vi "Update Outputs (Speed Controlled).vi"() -> ()   [LabVIEW 2012]
uses:
  Robot Global Data.vi
  <vilib>/addons/control/pid/NI_PID_pid.lvlib
  <vilib>/Rock Robotics/WPI/Solenoid/WPI_SolenoidSetEnum.vi
  <vilib>/Rock Robotics/WPI/Solenoid/WPI_SolenoidValue.ctl
  <vilib>/Rock Robotics/WPI/RobotDrive/WPI_RobotDriveArcadeDrive_Standard(NoSaturation).vi
  <vilib>/addons/control/pid/pid.llb/PID (DBL).vi
panel:
  out "Loop Time 2":u32(graph)
  out "Right Distance (ft)":dbl
  out "Left Distance (ft)":dbl
  out "Right Rate":dbl(graph)
  out "Left Rate":dbl(graph)
  in  "Shooter Speed (no encoder)":dbl(slide)=0.5 scale=0.0..1.0
  in  "Reset?":bool
  out "Shooter Output":dbl
  out "Loop Time":u32
  out "Rate":dbl
  out "Wheel Rate":dbl(graph)
  in  "Bang-Bang Output Range":T1={"Maximum"=1.0, "Minimum (Probably 0)"=0.0}
  in  "Bang-Bang Deadband Size":dbl=1.0
  in  "PID Output Range":cluster{"output high":dbl, "output low":dbl}={"output high"=1.0, "output low"=0.0} {"output low" format="%.2f"; "output high" format="%.2f"}
  in  "Shooter PID Gains":T2={"proportional gain (Kc)"=1.0, "integral time (Ti, min)"=0.01, "derivative time (Td, min)"=0.0} {"derivative time (Td, min)" format="%.3f"; "integral time (Ti, min)" format="%.3f"; "proportional gain (Kc)" format="%.3f"}
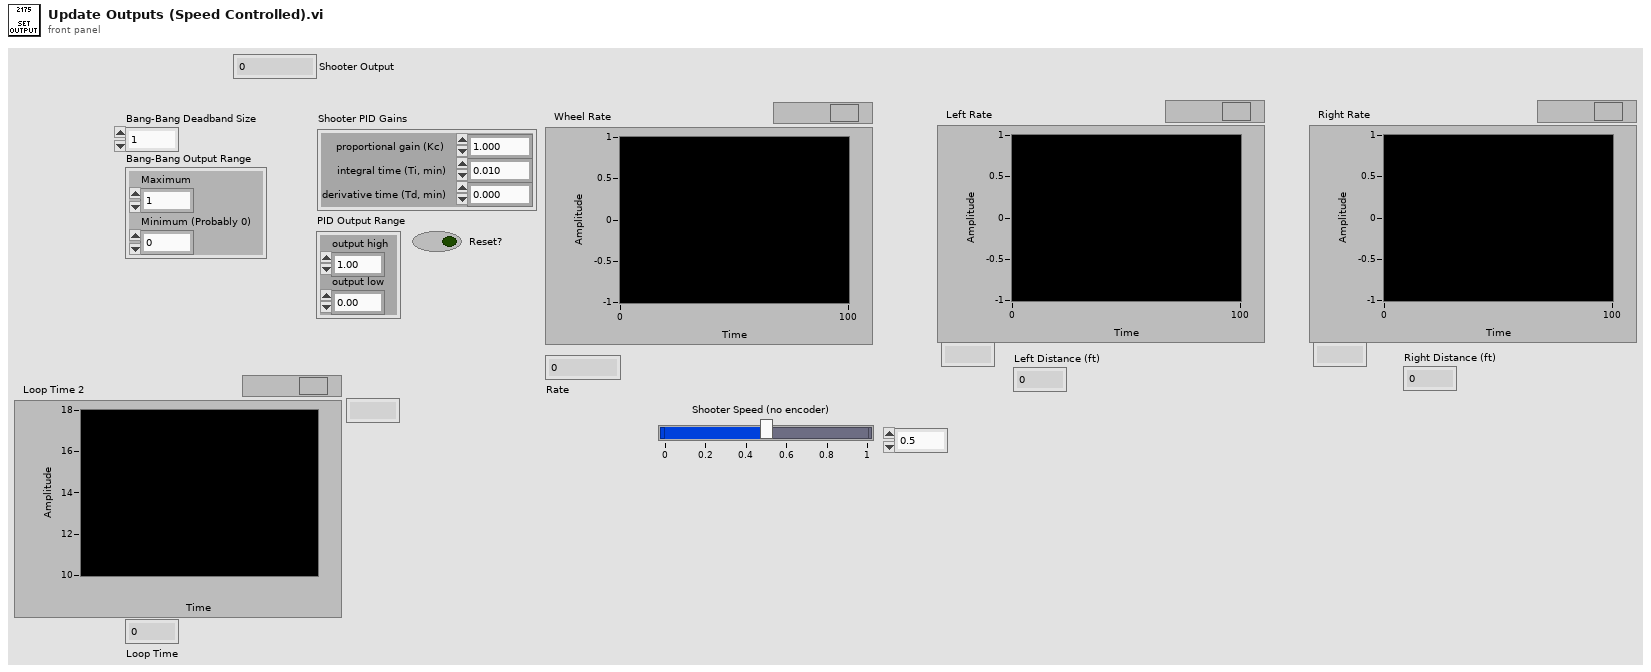
[diagram p1: front panel]
types:
  T1 = cluster{"Maximum":dbl, "Minimum (Probably 0)":dbl}
  T2 = cluster{"proportional gain (Kc)":dbl, "integral time (Ti, min)":dbl, "derivative time (Td, min)":dbl}
  T3 = typedef "WPI_SolenoidDevRef.ctl" = cluster{"DevStatus":errorcluster, "Solenoid Module":T4, "Forward Solenoid Channel":T5, "Reverse Solenoid Channel":T5}
  T4 = typedef "FPGA_TypedefSolenoidModule.ctl" = enum16{"Solenoid Module 1", "Solenoid Module 2"}
  T5 = typedef "WPI_SolenoidChannel.ctl" = enum8{"Solenoid 1", "Solenoid 2", "Solenoid 3", "Solenoid 4", "Solenoid 5", "Solenoid 6", "Solenoid 7", "Solenoid 8", "Invalid"}
  T6 = typedef "WPI_RobotDriveDevRef.ctl" = cluster{"DevStatus":errorcluster, "Motors[]":T7[], "Square Inputs":bool, "Max Output":dbl, "Isochronous":bool}
  T7 = typedef "WPI_MotorControlDeviceRef.ctl" = cluster{"DeviceStatus":errorcluster, "Type":enum16{"PWM", "CAN"}, "PWM":cluster{"Digital Module":T8, "PWM Channel":T9, "DeadBand":T10}, "CAN":cluster{"Device Number":u8, "Control Mode":T11, "Semaphore":T12, "Max Vout":dbl}, "Invert":bool, "TransformRef":T13, "InvTransformRef":T13}
  T8 = typedef "FPGA_TypedefDigitalModule.ctl" = enum16{"Digital Module 1", "Digital Module 2"}
  T9 = typedef "FPGA_DIOPWMChannel.ctl" = enum8{"PWM 1", "PWM 2", "PWM 3", "PWM 4", "PWM 5", "PWM 6", "PWM 7", "PWM 8", "PWM 9", "PWM 10", "Invalid"}
  T10 = typedef "WPI_PWMDeadband.ctl" = cluster{"Name":string, "maxPositivePwm":i32, "minPositivePwm":i32, "centerPwm":i32, "maxNegativePwm":i32, "minNegativePwm":i32, "angularRange":u16}
  T11 = typedef "WPI_CANJaguar_ControlMode.ctl" = enum8{"Percent VBus", "Current", "Speed", "Position", "Voltage"}
  T12 = typedef "Semaphore RefNum" = refnum<k1>
  T13 = typedef "WPI_PWMTransform_ConPane.ctl" = refnum<vi>
  T14 = typedef "WPI_DigitalInputDevRef.ctl" = cluster{"DevStatus":errorcluster, "DIO Channel":T15, "Digital Module":T8}
  T15 = typedef "FPGA_DIOChannel.ctl" = enum8{"DIO 1", "DIO 2", "DIO 3", "DIO 4", "DIO 5", "DIO 6", "DIO 7", "DIO 8", "DIO 9", "DIO 10", "DIO 11", "DIO 12", "DIO 13", "DIO 14", "Invalid"}
  T16 = typedef "WPI_EncoderDevRef.ctl" = cluster{"DevStatus":errorcluster, "EncoderIndex":T17, "CounterIndex":T18, "DistancePerCount":dbl, "Decoding Type":T19}
  T17 = typedef "FPGA_EncoderIdx.ctl" = enum8{"Enc 0", "Enc 1", "Enc 2", "Enc 3", "Invalid"}
  T18 = typedef "FPGA_CounterCtrSystemIndex.ctl" = enum8{"Ctr 0", "Ctr 1", "Ctr 2", "Ctr 3", "Ctr 4", "Ctr 5", "Ctr 6", "Ctr 7", "Invalid"}
  T19 = typedef "WPI_EncoderType.ctl" = enum16{"1x", "2x", "4x"}
  T20 = typedef "WPI_SolenoidValue.ctl" = enum16{"Off", "On", "Forward", "Reverse"}
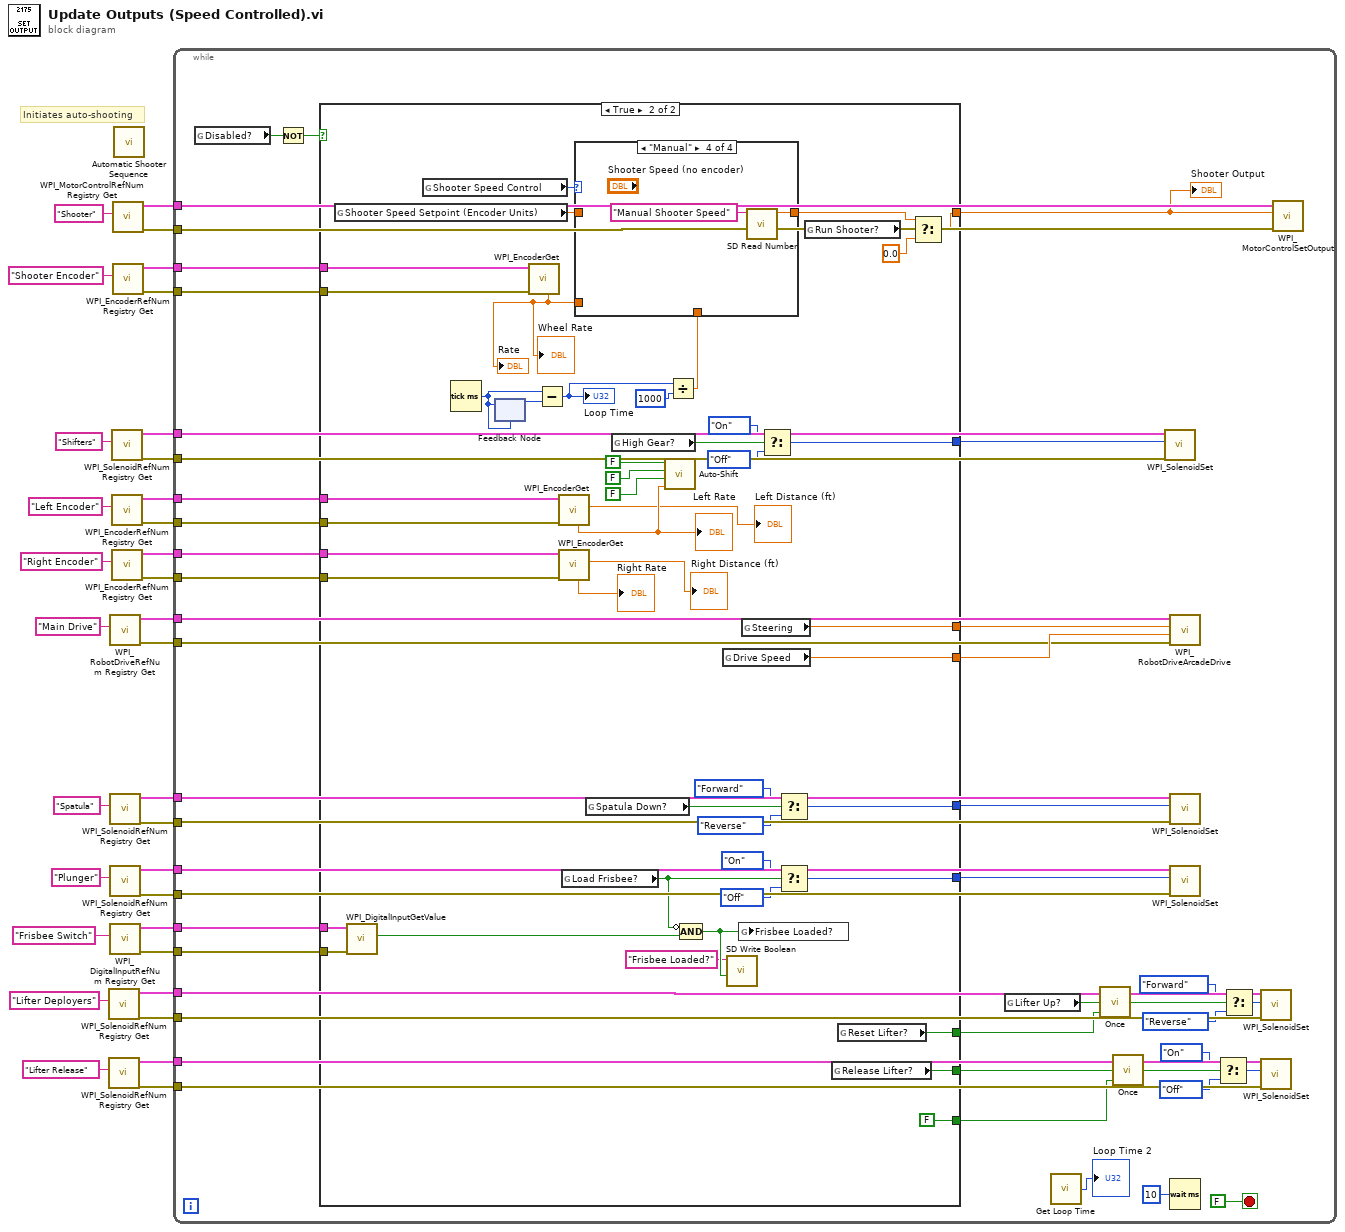
[diagram p0: block diagram]
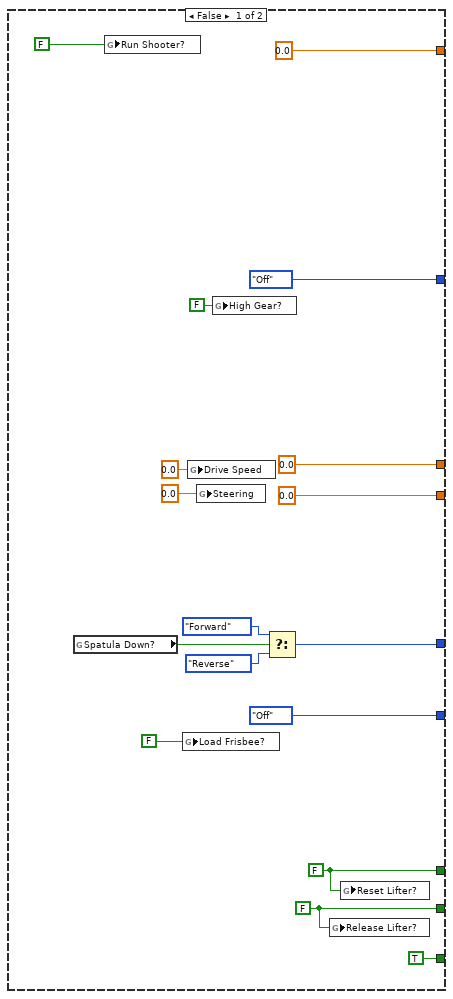
[diagram p2: hidden frame]
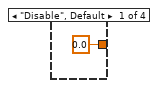
[diagram p3: hidden frame]
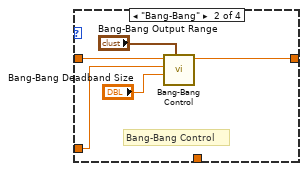
[diagram p4: hidden frame]
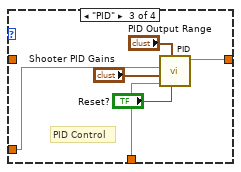
[diagram p5: hidden frame]
diagram:
  # "Initiates auto-shooting"
  n1 = call <vilib>:"WPI_SolenoidRefNum Registry Get.vi"("refnum name"="Lifter Deployers") -> ("error out"=w4:errorcluster, "SolenoidDevRef"=w5:T3)  [unwired: 9 in]
  n2 = call <vilib>:"WPI_SolenoidRefNum Registry Get.vi"("refnum name"="Lifter Release") -> ("error out"=w3:errorcluster, "SolenoidDevRef"=w2:T3)  [unwired: 9 in]
  n3 = call <vilib>:"WPI_RobotDriveRefNum Registry Get.vi"("refnum name"="Main Drive") -> ("error out"=w25:errorcluster, "RobotDriveDevRef"=w26:T6)  [unwired: 9 in]
  n4 = call <vilib>:"WPI_SolenoidRefNum Registry Get.vi"("refnum name"="Spatula") -> ("error out"=w19:errorcluster, "SolenoidDevRef"=w20:T3)  [unwired: 9 in]
  n5 = call <vilib>:"WPI_SolenoidRefNum Registry Get.vi"("refnum name"="Plunger") -> ("error out"=w18:errorcluster, "SolenoidDevRef"=w17:T3)  [unwired: 9 in]
  n6 = call <vilib>:"WPI_DigitalInputRefNum Registry Get.vi"("refnum name"="Frisbee Switch") -> ("error out"=w7:errorcluster, "DigitalInputDevRef"=w8:T14)  [unwired: 9 in]
  n7 = call <vilib>:"WPI_SolenoidRefNum Registry Get.vi"("refnum name"="Shifters") -> ("error out"=w22:errorcluster, "SolenoidDevRef"=w23:T3)  [unwired: 9 in]
  n8 = call <vilib>:"WPI_EncoderRefNum Registry Get.vi"("refnum name"="Left Encoder") -> ("error out"=w13:errorcluster, "EncoderDevRef"=w14:T16)  [unwired: 9 in]
  n9 = call <vilib>:"WPI_EncoderRefNum Registry Get.vi"("refnum name"="Right Encoder") -> ("error out"=w12:errorcluster, "EncoderDevRef"=w11:T16)  [unwired: 9 in]
  n10 = call <vilib>:"WPI_MotorControlRefNum Registry Get.vi"("refnum name"="Shooter") -> ("error out"=w28:errorcluster, "MotorControlDevRef"=w29:T7)  [unwired: 9 in]
  n11 = call <vilib>:"WPI_EncoderRefNum Registry Get.vi"("refnum name"="Shooter Encoder") -> ("error out"=w30:errorcluster, "EncoderDevRef"=w31:T16)  [unwired: 9 in]
  n12 = call "Automatic Shooter Sequence.vi"() -> ()  [unwired: 12 in]
  n13 = while {
    tunnel: w31 -> [w74]
    tunnel: w30 -> [w73]
    tunnel: w29 -> [w72]
    tunnel: w28 -> [w71]
    tunnel: w26 -> [w68]
    tunnel: w25 -> [w67]
    tunnel: w23 -> [w66]
    tunnel: w22 -> [w65]
    tunnel: w20 -> [w62]
    tunnel: w19 -> [w63]
    tunnel: w17 -> [w61]
    tunnel: w18 -> [w60]
    tunnel: w14 -> [w56]
    tunnel: w13 -> [w55]
    tunnel: w11 -> [w53]
    tunnel: w12 -> [w54]
    tunnel: w8 -> [w52]
    tunnel: w7 -> [w51]
    tunnel: w5 -> [w50]
    tunnel: w4 -> [w49]
    tunnel: w2 -> [w48]
    tunnel: w3 -> [w47]
    stop <- FALSE stop-if-true
    n14 = global read "Robot Global Data.vi" "Disabled?"() -> (w76:bool)
    n15 = Not(x=w76) -> (.not. x?=w75:bool)
    n16 = case shown="True" w75 {
      tunnel: w74 -> [_ w142]
      tunnel: w73 -> [_ w141]
      tunnel: [0.0 ("Output") w112] -> w57
      tunnel: [0.0 ("Steering") w140] -> w70
      tunnel: [0.0 ("Drive Speed") w121] -> w69
      tunnel: [w86 w127] -> w64
      tunnel: [WPI_SolenoidValue."Off" ("Value") w123] -> w59
      tunnel: [WPI_SolenoidValue."Off" ("Value") w119] -> w58
      tunnel: w56 -> [_ w117]
      tunnel: w55 -> [_ w116]
      tunnel: w53 -> [_ w108]
      tunnel: w54 -> [_ w109]
      tunnel: w52 -> [_ w104]
      tunnel: w51 -> [_ w103]
      tunnel: [w81 w98] -> w41
      tunnel: [TRUE ("High Gear?") FALSE ("High Gear?")] -> w40
      tunnel: [w79 w96] -> w34
      frame False {
        w79 = FALSE ("High Gear?")
        w81 = FALSE ("High Gear?")
        n17 = global read "Robot Global Data.vi" "Spatula Down?"() -> (w87:bool)
        n18 = global write "Robot Global Data.vi" "Run Shooter?"(FALSE ("High Gear?")) -> ()
        n19 = global write "Robot Global Data.vi" "Load Frisbee?"(FALSE ("High Gear?")) -> ()
        n20 = global write "Robot Global Data.vi" "Drive Speed"(0.0 ("Shooter Speed")) -> ()
        n21 = global write "Robot Global Data.vi" "Steering"(0.0 ("Shooter Speed")) -> ()
        n22 = global write "Robot Global Data.vi" "High Gear?"(FALSE ("High Gear?")) -> ()
        n23 = Select(t=WPI_SolenoidValue."Forward" ("Value"), s=w87, f=WPI_SolenoidValue."Reverse" ("Value")) -> (s? t:f=w86:T20)
        n24 = global write "Robot Global Data.vi" "Release Lifter?"(w81) -> ()
        n25 = global write "Robot Global Data.vi" "Reset Lifter?"(w79) -> ()
      }
      frame True {
        n26 = global read "Robot Global Data.vi" "Shooter Speed Setpoint (Encoder Units)"() -> (w129:dbl)
        n27 = call <vilib>:"WPI_DigitalInputGetValue.vi"("error in (no error)"=w103, "DigitalInputDevRef"=w104) -> ("Value"=w102:bool)  [unwired: 7 in, 2 out]
        n28 = global read "Robot Global Data.vi" "Shooter Speed Control"() -> (w115:enum16{"Disable", "Bang-Bang", "PID", "Manual"})
        n29 = Tick Count (ms)() -> (millisecond timer value=w138:u32)
        n30 = feedback-in #1(w138) -> ()
        n31 = feedback #1(w138) -> (w139:u32)
        n32 = call <vilib>:"WPI_EncoderGet.vi"("error in (no error)"=w141, "EncoderDevRef"=w142) -> ("Rate"=w130:dbl)  [unwired: 4 in, 5 out]
        "Wheel Rate" <- w130
        "Rate" <- w130
        n33 = Subtract(x=w138, y=w139) -> (x-y=w137:u32)
        "Loop Time" <- w137
        n34 = call <vilib>:"WPI_EncoderGet.vi"("error in (no error)"=w116, "EncoderDevRef"=w117) -> ("Distance"=→"Left Distance (ft)":dbl, "Rate"=w110:dbl)  [unwired: 4 in, 4 out]
        "Left Rate" <- w110
        n35 = call <vilib>:"WPI_EncoderGet.vi"("error in (no error)"=w109, "EncoderDevRef"=w108) -> ("Distance"=→"Right Distance (ft)":dbl, "Rate"=→"Right Rate":dbl)  [unwired: 4 in, 4 out]
        n36 = global read "Robot Global Data.vi" "Load Frisbee?"() -> (w101:bool)
        n37 = global read "Robot Global Data.vi" "Spatula Down?"() -> (w125:bool)
        n38 = global read "Robot Global Data.vi" "High Gear?"() -> (w134:bool)
        n39 = call "Auto-Shift.vi"("Average Ft/Sec"=w110, "Coastdown Enabled?"=FALSE, "Kickdown Enabled?"=FALSE, "Upshift Enabled?"=FALSE) -> ()  [unwired: 1 in]
        n40 = Divide(x=w137, y=u32 1000) -> (x/y=w135:dbl)
        n41 = case shown="\"Manual\"" w115 {
          tunnel: w130 -> [_ w148 w154 _]
          tunnel: [0.0 ("Output") w145 w153 w156] -> w113
          tunnel: w129 -> [_ w144 _ _]
          tunnel: w135 -> [_ _ w152 _]
          frame "Disable", Default {
          }
          frame "Bang-Bang" {
            # "Bang-Bang Control"
            n42 = call "Bang-Bang Control.vi"("Output Range"="Bang-Bang Output Range", "Deadband Size"="Bang-Bang Deadband Size", "Process Variable"=w148, "Setpoint"=w144) -> ("Output"=w145:dbl)  [unwired: 7 in]
          }
          frame "PID" {
            # "PID Control"
            n43 = call-poly <vilib>:"PID.vi"("reinitialize? (F)"="Reset?", "output range"="PID Output Range", "dt (s)"=w152, "PID gains"="Shooter PID Gains", "process variable"=w154) -> ("output"=w153:dbl)  [unwired: 5 in, 1 out]
          }
          frame "Manual" {
            n44 = call <vilib>:"SD Read Number.vi"("Name"="Manual Shooter Speed") -> ("Numeric"=w156:dbl)  [unwired: 8 in, 2 out]
          }
        }
        n45 = Compound Arithmetic op=AND(invert w101, w102) -> (w100:bool)
        n46 = global read "Robot Global Data.vi" "Drive Speed"() -> (w121:dbl)
        n47 = call <vilib>:"SD Write Boolean.vi"("Boolean"=w100, "Name"="Frisbee Loaded?") -> ()  [unwired: 8 in, 2 out]
        n48 = global write "Robot Global Data.vi" "Frisbee Loaded?"(w100) -> ()
        n49 = global read "Robot Global Data.vi" "Steering"() -> (w140:dbl)
        n50 = Select(t=WPI_SolenoidValue."On" ("Value"), s=w134, f=WPI_SolenoidValue."Off" ("Value")) -> (s? t:f=w119:T20)
        n51 = Select(t=WPI_SolenoidValue."Forward" ("Value"), s=w125, f=WPI_SolenoidValue."Reverse" ("Value")) -> (s? t:f=w127:T20)
        n52 = Select(t=WPI_SolenoidValue."On" ("Value"), s=w101, f=WPI_SolenoidValue."Off" ("Value")) -> (s? t:f=w123:T20)
        n53 = global read "Robot Global Data.vi" "Run Shooter?"() -> (w114:bool)
        n54 = global read "Robot Global Data.vi" "Release Lifter?"() -> (w98:bool)
        n55 = global read "Robot Global Data.vi" "Reset Lifter?"() -> (w96:bool)
        n56 = Select(t=w113, s=w114, f=0.0) -> (s? t:f=w112:dbl)
      }
    }
    "Shooter Output" <- w57
    n57 = global read "Robot Global Data.vi" "Lifter Up?"() -> (w36:bool)
    n58 = call "Get Loop Time.vi"() -> ("Loop Time"=→"Loop Time 2":u32)  [unwired: 1 in]
    n59 = call "Once.vi"("Reset?"=w34, "Input"=w36) -> ("Output"=w35:bool)  [unwired: 1 in]
    n60 = call "Once.vi"("Reset?"=w40, "Input"=w41) -> ("Output"=w42:bool)  [unwired: 1 in]
    n61 = call-poly <vilib>:"WPI_SolenoidSet.vi"("error in (no error)"=w65, "Value"=w58, "SolenoidDevRef"=w66) -> ()  [unwired: 7 in, 2 out]
    n62 = call-poly <vilib>:"WPI_RobotDriveArcadeDrive.vi"("error in (no error)"=w67, "Y axis value"=w69, "X axis value"=w70, "RobotDriveDevRef"=w68) -> ()  [unwired: 5 in, 3 out]
    n63 = call-poly <vilib>:"WPI_SolenoidSet.vi"("error in (no error)"=w63, "Value"=w64, "SolenoidDevRef"=w62) -> ()  [unwired: 7 in, 2 out]
    n64 = call-poly <vilib>:"WPI_SolenoidSet.vi"("error in (no error)"=w60, "Value"=w59, "SolenoidDevRef"=w61) -> ()  [unwired: 7 in, 2 out]
    n65 = Wait (ms)(milliseconds to wait=u32 10) -> ()  [unwired: 1 out]
    n66 = Select(t=WPI_SolenoidValue."On" ("Value"), s=w42, f=WPI_SolenoidValue."Off" ("Value")) -> (s? t:f=w43:T20)
    n67 = Select(t=WPI_SolenoidValue."Forward" ("Value"), s=w35, f=WPI_SolenoidValue."Reverse" ("Value")) -> (s? t:f=w37:T20)
    n68 = call-poly <vilib>:"WPI_SolenoidSet.vi"("error in (no error)"=w49, "Value"=w37, "SolenoidDevRef"=w50) -> ()  [unwired: 7 in, 2 out]
    n69 = call-poly <vilib>:"WPI_SolenoidSet.vi"("error in (no error)"=w47, "Value"=w43, "SolenoidDevRef"=w48) -> ()  [unwired: 7 in, 2 out]
    n70 = call <vilib>:"WPI_MotorControlSetOutput.vi"("error in (no error)"=w71, "Output"=w57, "MotorControlDevRef"=w72) -> ()  [unwired: 6 in, 3 out]
  }
